vi "Mobility Calculator.vi"() -> ()   [LabVIEW 2011]
uses:
  <vilib>/picture/picture.llb/Draw True-Color Pixmap.vi
panel:
  in  "Blank Button":bool
  in  "Refresh Button":bool
  in  "tick mark length":i16=4
  in  "constant coordinate":i16=10
  out "picture":picture
  in  "scale definition":T1={"coordinate 1"=5, "value 1"=0.0, "coordinate 2"=50, "value 2"=10.0, "log"=FALSE, "fmt and prec"={"format"=enum."Decimal", "precision"=0}} {"value 2" format="%0.2f"; "value 1" format="%0.2f"}
  in  "scale attributes":T2={"horizontal"=FALSE, "left/top"=FALSE, "draw bar"=TRUE, "line color"=255, "text color"=0}
  out "2D Picture 2":picture
  out "Array 6":dbl[][](array[numeric])
  out "Cluster":T3
  out "Array 5":dbl[](array[numeric])
  out "Array 4":dbl[](array[numeric])
  out "Array 3":dbl[](array[numeric])
  out "Numeric 2":dbl
  out "Numeric":dbl
  out "2D Picture":picture
  in  "Path 3":path
  in  "Slide":dbl(slide) step=1.0 scale=-1.0..142.0 scale format="%#_1p"
  out "New Mobility":dbl
  out "Array 2":dbl[](array[numeric])
  out "Array":dbl[](array[numeric])
  in  "Width new":dbl
  in  "Length new":dbl
  in  "Dielectric (d) new":dbl
  in  "Save Changes?":bool
  out "Index":dbl
  out "String":string
  in  "Path 2":path
  in  "Down Button":bool
  in  "Up Button":bool
  in  "Previous Button":bool
  in  "Next Button":bool
  in  "Cancel Button":bool
  in  "NumPts":dbl=5.0
  out "XY Graph":cluster{dbl[], dbl[]}[](graph)
  out "Dielectric (d)":dbl
  out "Width":dbl
  out "Length":dbl
  out "Table Control 2":string[][](table)
  out "Table Control":string[][](table)
  in  "Row Start":dbl=20.0
  in  "Path":path
  out "Mobility":dbl
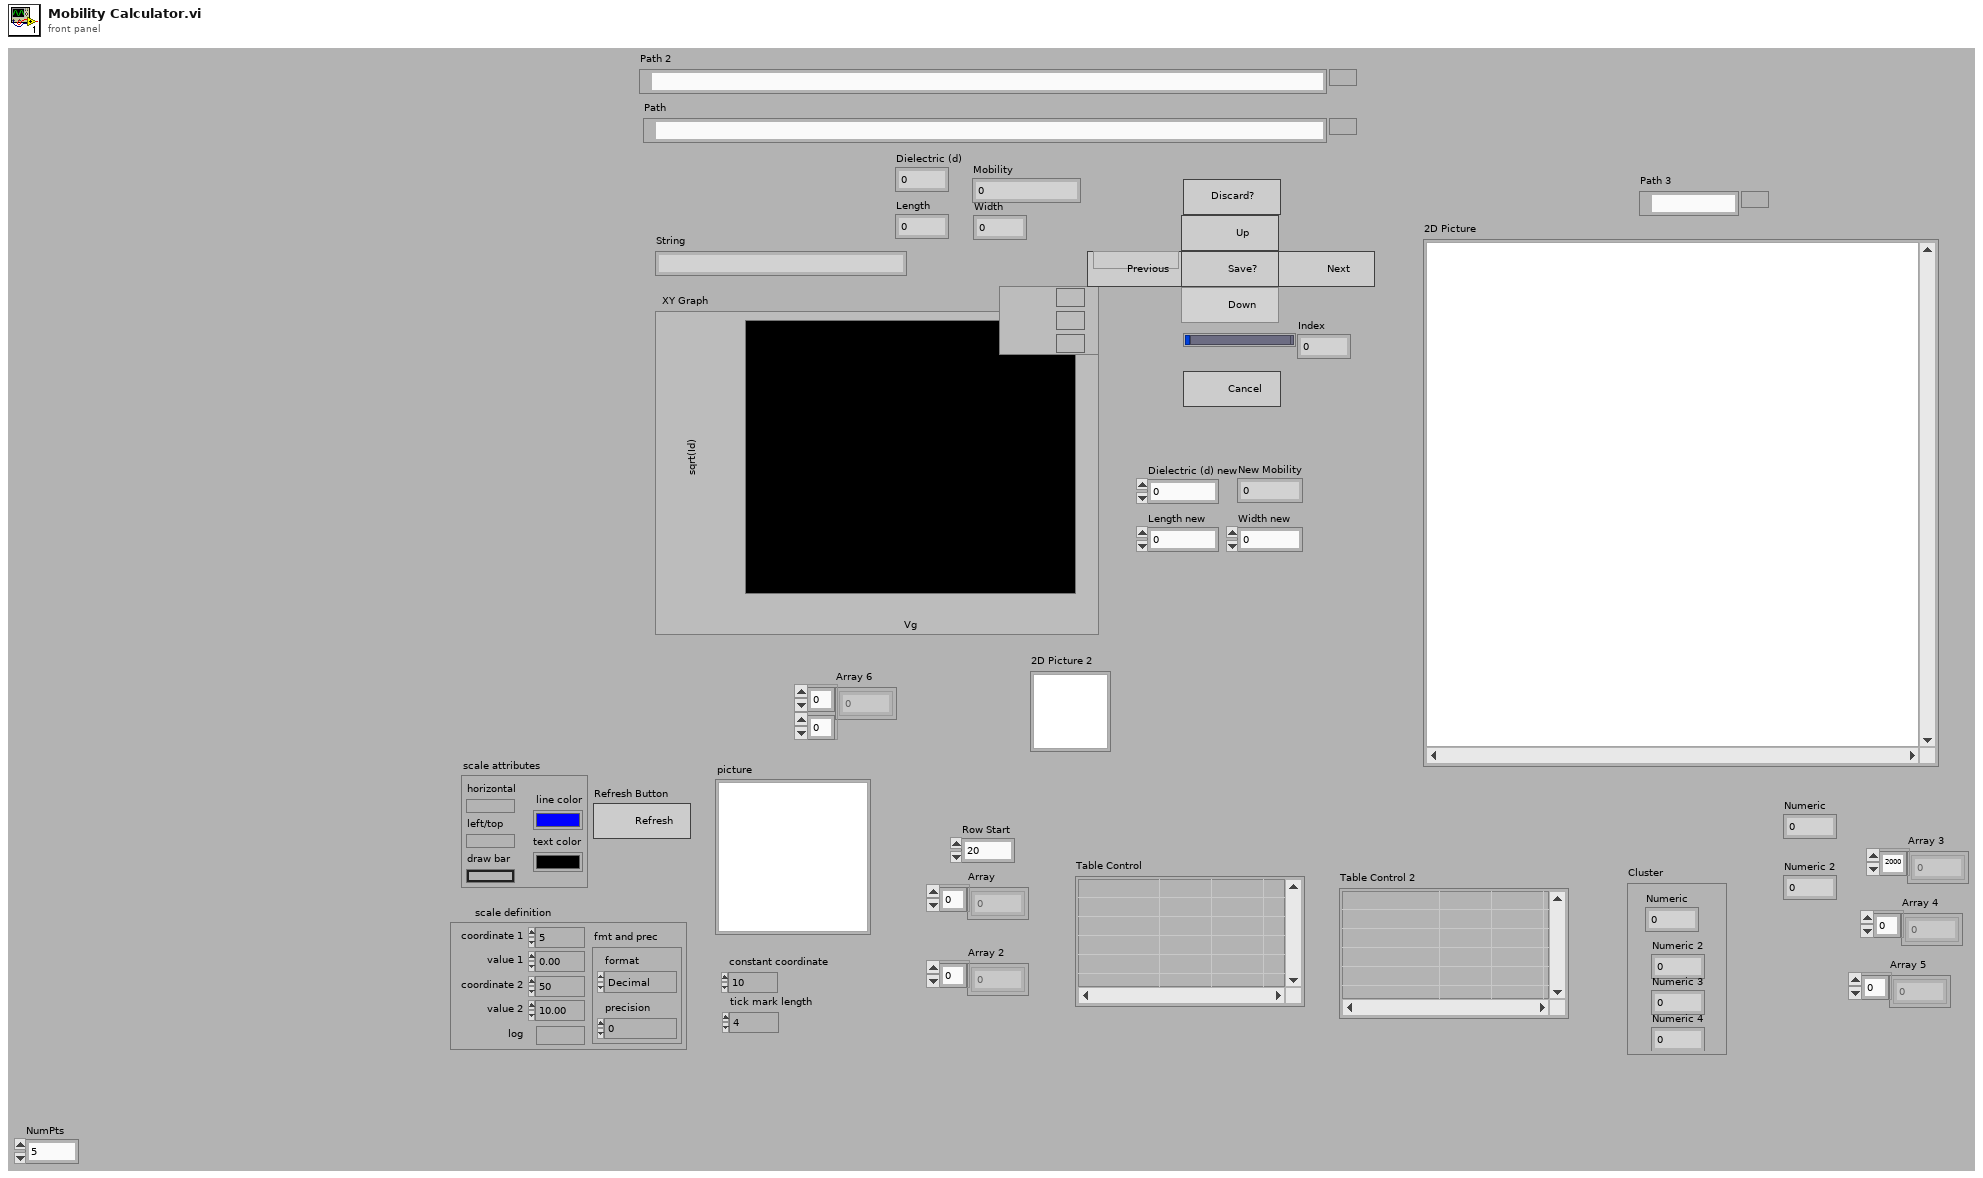
[diagram p1: front panel]
types:
  T1 = cluster{"coordinate 1":i16, "value 1":dbl, "coordinate 2":i16, "value 2":dbl, "log":bool, "fmt and prec":cluster{"format":enum8{"Decimal", "Scientific", "Engineering", "Binary", "Octal", "Hex"}, "precision":u8}}
  T2 = cluster{"horizontal":bool, "left/top":bool, "draw bar":bool, "line color":u32, "text color":u32}
  T3 = cluster{"Numeric":dbl, "Numeric 2":dbl, "Numeric 3":dbl, "Numeric 4":dbl}
  T4 = cluster{"[0]":cluster{dbl[], dbl[]}, "[1]":cluster{dbl[], dbl[]}, "[2]":cluster{dbl[], dbl[]}, "[3]":cluster{dbl[], dbl[]}, "[4]":cluster{dbl[], dbl[]}, "[5]":cluster{dbl[], dbl[]}, "[6]":cluster{dbl[], dbl[]}, "[7]":cluster{dbl[], dbl[]}, "[8]":cluster{dbl[], dbl[]}}
  T5 = typedef "imagedata.ctl" = cluster{"image type":i32, "image depth":i32, "image":u8[], "mask":u8[], "colors":u32[], "Rectangle":cluster{"left":i16, "top":i16, "right":i16, "bottom":i16}}
  T6 = cluster{"left":i16, "top":i16, "right":i16, "bottom":i16}
  T7 = cluster{"image type":i32, "image depth":i32, "image":u8[], "mask":u8[], "colors":u32[], cluster{dbl, dbl, dbl, dbl}}
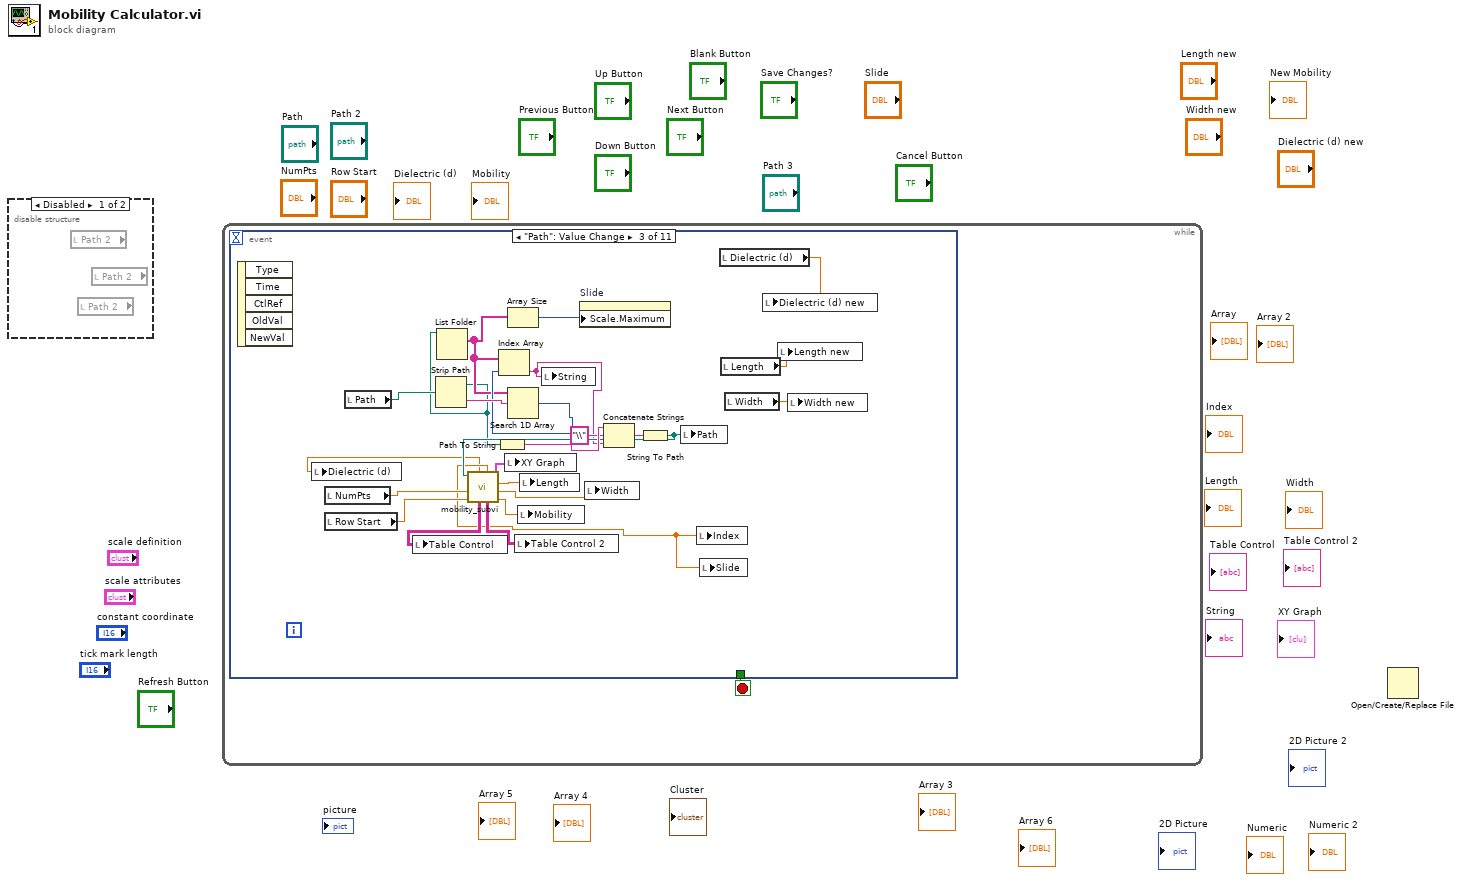
[diagram p0: block diagram]
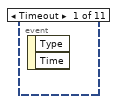
[diagram p3: hidden frame]
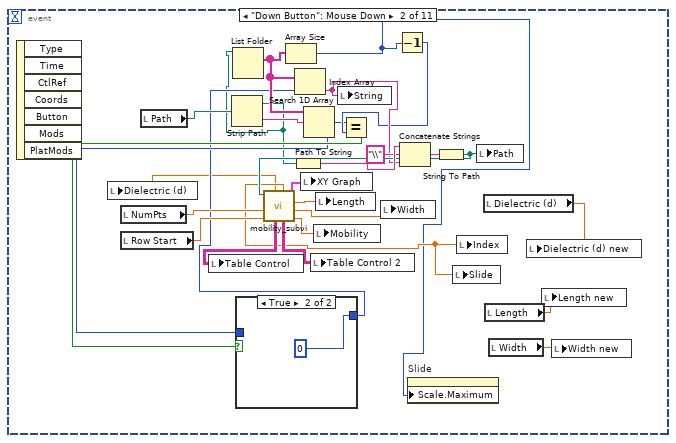
[diagram p4: hidden frame]
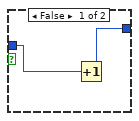
[diagram p5: hidden frame]
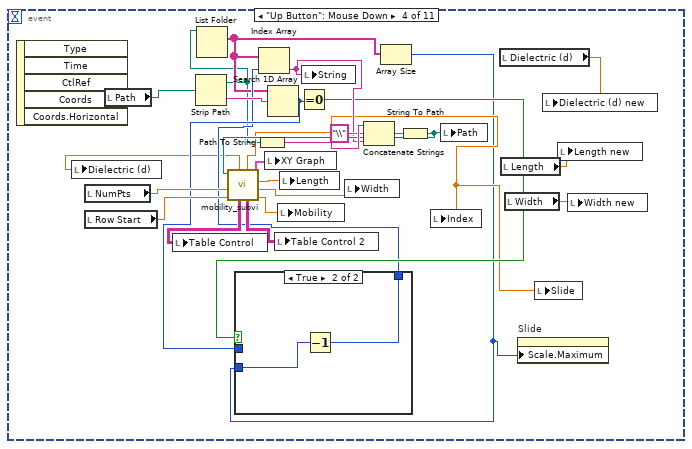
[diagram p6: hidden frame]
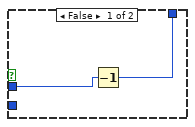
[diagram p7: hidden frame]
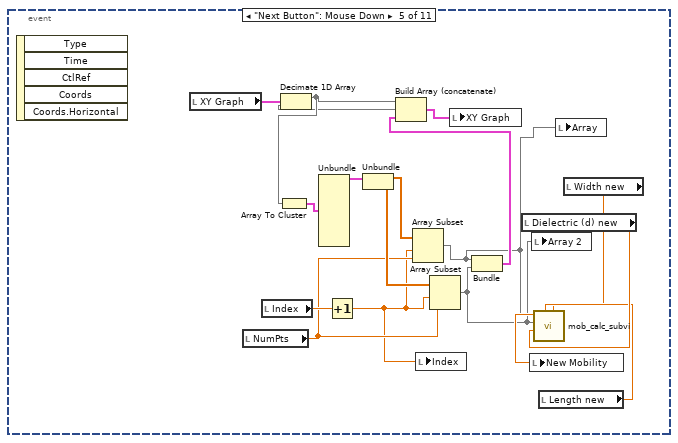
[diagram p8: hidden frame]
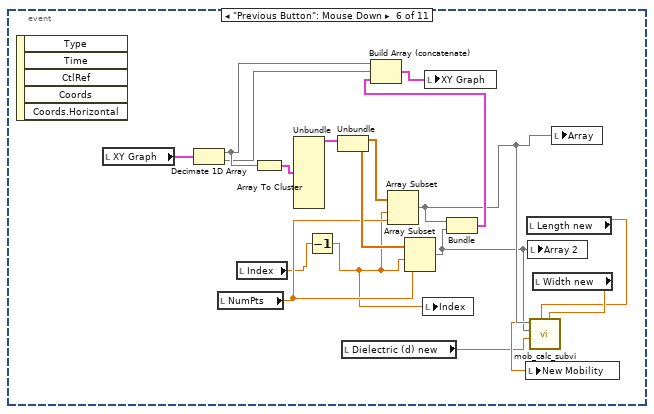
[diagram p9: hidden frame]
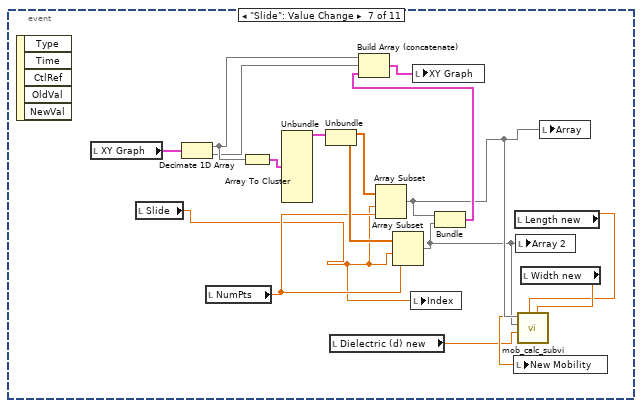
[diagram p10: hidden frame]
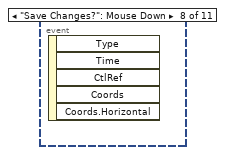
[diagram p11: hidden frame]
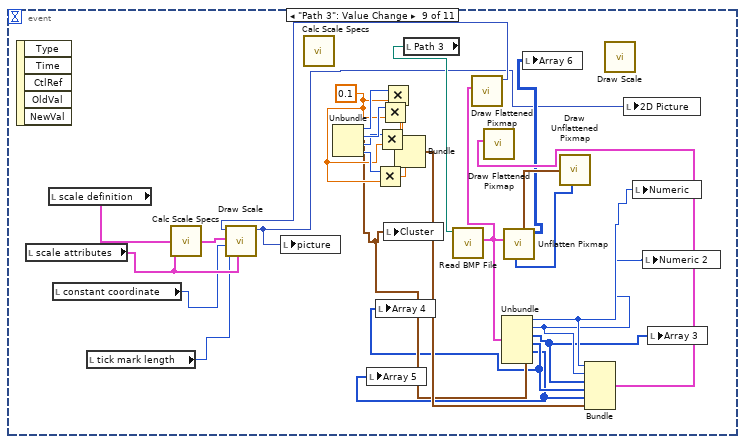
[diagram p12: hidden frame]
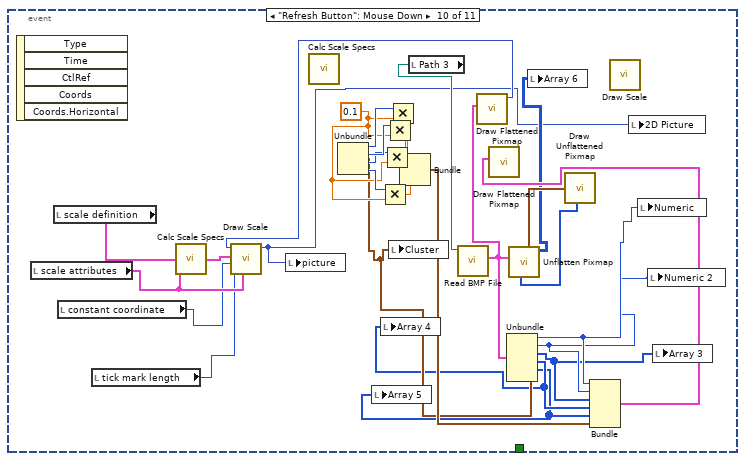
[diagram p13: hidden frame]
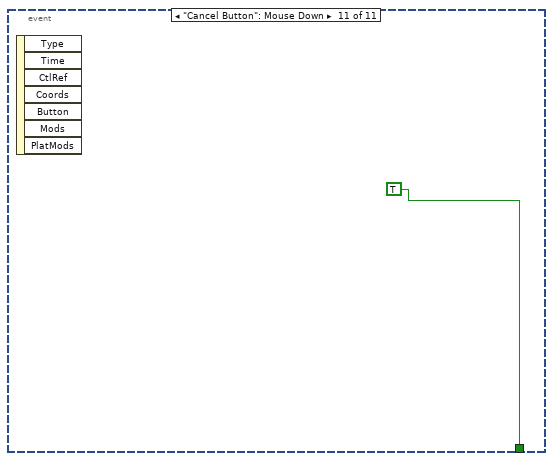
[diagram p14: hidden frame]
diagram:
  n1 = disable-structure shown="Disabled" {
    frame Disabled {
      n2 = local read "Path 2"() -> ()  [unwired: 1 out]
      n3 = local read "Path 2"() -> ()  [unwired: 1 out]
      n4 = local read "Path 2"() -> ()  [unwired: 1 out]
    }
    frame Enabled {
    }
  }
  n5 = while {
    stop <- w1 stop-if-true
    n6 = event shown="[2] \"Path\": Value Change" {
      selector: _ -> [_ _ _ _ _ _ _ _ _ _ _]
      dyn-events: _ -> [_ _ _ _ _ _ _ _ _ _ _]
      timeout: _ -> [_ _ _ _ _ _ _ _ _ _ _]
      tunnel: [_ _ _ _ _ _ _ _ _ _ TRUE] -> w1
      event Timeout {
        n7 = event-data() -> ()  [unwired: 1 in, 2 out]
      }
      event "Down Button": Mouse Down {
        n8 = event-data() -> ()  [unwired: 1 in, 7 out]
        n9 = local read "NumPts"() -> (w22:dbl)
        n10 = local read "Row Start"() -> (w21:dbl)
        n11 = local read "Path"() -> (w28:path)
        n12 = Strip Path(path=w28) -> (stripped path=w2:path, name=w26:string)
        n13 = List Folder(path=w2) -> (filenames=w13:string[])  [unwired: 3 in, 3 out]
        n14 = Array Size(array=w13) -> (size(s)=w4:i32)
        n15 = Path To String(path=w2) -> (string=w27:string)
        n16 = Search 1D Array(1D array=w13, element=w26) -> (index of element=w10:i32)  [unwired: 1 in]
        n17 = Decrement(x=w4) -> (x-1=w11:i32)
        n18 = Equal?(x=w10, y=w11) -> (x = y?=w12:bool)
        n19 = case shown="True" w12 {
          tunnel: w10 -> [w30 _]
          tunnel: [w29 0] -> w9
          frame False {
            n20 = Increment(x=w30) -> (x+1=w29:i32)
          }
          frame True {
          }
        }
        n21 = Index Array(array=w13, index=w9) -> (element=w14:string)
        n22 = local write "String"(w14) -> ()
        n23 = Concatenate Strings(w27, "\\", w14) -> (w25:string)
        n24 = property on="Slide" class="Slide (strict)"("Scale.Maximum"=w4) -> ()  [unwired: 2 in, 2 out]
        n25 = String To Path(string=w25) -> (path=w23:path)
        n26 = call "mobility_subvi.vi"("Row Start"=w21, "NumPts"=w22, "Path"=w23) -> ("Mobility"=w15:dbl, "Width"=w16:dbl, "Length"=w17:dbl, "XY Graph"=w18:cluster{dbl[], dbl[]}[], "Table Control 2"=w19:string[][], "Index"=w5:dbl, "Table Control"=w20:string[][], "Dielectric (d)"=w3:dbl)  [unwired: 1 in]
        n27 = local write "Dielectric (d)"(w3) -> ()
        n28 = local write "Table Control"(w20) -> ()
        n29 = local write "XY Graph"(w18) -> ()
        n30 = local write "Table Control 2"(w19) -> ()
        n31 = local write "Mobility"(w15) -> ()
        n32 = local write "Length"(w17) -> ()
        n33 = local write "Width"(w16) -> ()
        n34 = local write "Slide"(w5) -> ()
        n35 = local write "Index"(w5) -> ()
        n36 = local write "Path"(w23) -> ()
        n37 = local read "Dielectric (d)"() -> (w8:dbl)
        n38 = local read "Length"() -> (w7:dbl)
        n39 = local read "Width"() -> (w6:dbl)
        n40 = local write "Dielectric (d) new"(w8) -> ()
        n41 = local write "Length new"(w7) -> ()
        n42 = local write "Width new"(w6) -> ()
      }
      event "Path": Value Change {
        n43 = event-data() -> ()  [unwired: 1 in, 5 out]
        n44 = local read "NumPts"() -> (w49:dbl)
        n45 = local read "Row Start"() -> (w48:dbl)
        n46 = local read "Path"() -> (w55:path)
        n47 = Strip Path(path=w55) -> (stripped path=w32:path, name=w53:string)
        n48 = List Folder(path=w32) -> (filenames=w35:string[])  [unwired: 3 in, 3 out]
        n49 = Path To String(path=w32) -> (string=w54:string)
        n50 = Array Size(array=w35) -> (size(s)=w34:i32)
        n51 = Search 1D Array(1D array=w35, element=w53) -> (index of element=w40:i32)  [unwired: 1 in]
        n52 = Index Array(array=w35, index=w40) -> (element=w41:string)
        n53 = local write "String"(w41) -> ()
        n54 = property on="Slide" class="Slide (strict)"("Scale.Maximum"=w34) -> ()  [unwired: 2 in, 2 out]
        n55 = Concatenate Strings(w54, "\\", w41) -> (w52:string)
        n56 = String To Path(string=w52) -> (path=w50:path)
        n57 = call "mobility_subvi.vi"("Row Start"=w48, "NumPts"=w49, "Path"=w50) -> ("Mobility"=w42:dbl, "Width"=w43:dbl, "Length"=w44:dbl, "XY Graph"=w45:cluster{dbl[], dbl[]}[], "Table Control 2"=w46:string[][], "Index"=w36:dbl, "Table Control"=w47:string[][], "Dielectric (d)"=w33:dbl)  [unwired: 1 in]
        n58 = local write "Dielectric (d)"(w33) -> ()
        n59 = local write "Table Control"(w47) -> ()
        n60 = local write "XY Graph"(w45) -> ()
        n61 = local write "Table Control 2"(w46) -> ()
        n62 = local write "Mobility"(w42) -> ()
        n63 = local write "Length"(w44) -> ()
        n64 = local write "Width"(w43) -> ()
        n65 = local write "Path"(w50) -> ()
        n66 = local write "Index"(w36) -> ()
        n67 = local write "Slide"(w36) -> ()
        n68 = local read "Dielectric (d)"() -> (w39:dbl)
        n69 = local read "Length"() -> (w38:dbl)
        n70 = local read "Width"() -> (w37:dbl)
        n71 = local write "Dielectric (d) new"(w39) -> ()
        n72 = local write "Length new"(w38) -> ()
        n73 = local write "Width new"(w37) -> ()
      }
      event "Up Button": Mouse Down {
        n74 = event-data() -> ()  [unwired: 1 in, 5 out]
        n75 = local read "NumPts"() -> (w75:dbl)
        n76 = local read "Row Start"() -> (w74:dbl)
        n77 = local read "Path"() -> (w81:path)
        n78 = Strip Path(path=w81) -> (stripped path=w56:path, name=w79:string)
        n79 = List Folder(path=w56) -> (filenames=w63:string[])  [unwired: 3 in, 3 out]
        n80 = Path To String(path=w56) -> (string=w80:string)
        n81 = Search 1D Array(1D array=w63, element=w79) -> (index of element=w65:i32)  [unwired: 1 in]
        n82 = Equal To 0?(x=w65) -> (x = 0?=w66:bool)
        n83 = Array Size(array=w63) -> (size(s)=w58:i32)
        n84 = case shown="True" w66 {
          tunnel: w65 -> [w83 _]
          tunnel: [w82 w84] -> w64
          tunnel: w58 -> [_ w85]
          frame False {
            n85 = Decrement(x=w83) -> (x-1=w82:i32)
          }
          frame True {
            n86 = Decrement(x=w85) -> (x-1=w84:i32)
          }
        }
        n87 = Index Array(array=w63, index=w64) -> (element=w67:string)
        n88 = local write "String"(w67) -> ()
        n89 = Concatenate Strings(w80, "\\", w67) -> (w78:string)
        n90 = String To Path(string=w78) -> (path=w76:path)
        n91 = call "mobility_subvi.vi"("Row Start"=w74, "NumPts"=w75, "Path"=w76) -> ("Mobility"=w68:dbl, "Width"=w69:dbl, "Length"=w70:dbl, "XY Graph"=w71:cluster{dbl[], dbl[]}[], "Table Control 2"=w72:string[][], "Index"=w59:dbl, "Table Control"=w73:string[][], "Dielectric (d)"=w57:dbl)  [unwired: 1 in]
        n92 = local write "Dielectric (d)"(w57) -> ()
        n93 = local write "Table Control"(w73) -> ()
        n94 = local write "XY Graph"(w71) -> ()
        n95 = local write "Table Control 2"(w72) -> ()
        n96 = local write "Mobility"(w68) -> ()
        n97 = local write "Length"(w70) -> ()
        n98 = local write "Width"(w69) -> ()
        n99 = local write "Index"(w59) -> ()
        n100 = local write "Path"(w76) -> ()
        n101 = local read "Dielectric (d)"() -> (w62:dbl)
        n102 = local read "Length"() -> (w61:dbl)
        n103 = local read "Width"() -> (w60:dbl)
        n104 = property on="Slide" class="Slide (strict)"("Scale.Maximum"=w58) -> ()  [unwired: 2 in, 2 out]
        n105 = local write "Slide"(w59) -> ()
        n106 = local write "Dielectric (d) new"(w62) -> ()
        n107 = local write "Length new"(w61) -> ()
        n108 = local write "Width new"(w60) -> ()
      }
      event "Next Button": Mouse Down {
        n109 = event-data() -> ()  [unwired: 1 in, 5 out]
        n110 = local read "XY Graph"() -> (w97:cluster{dbl[], dbl[]}[])
        n111 = local read "NumPts"() -> (w98:dbl)
        n112 = local read "Index"() -> (w99:dbl)
        n113 = Decimate 1D Array(w97) -> (w93:cluster{dbl[], dbl[]}[], w92:cluster{dbl[], dbl[]}[])
        n114 = Array To Cluster(array=w93) -> (cluster=w103:T4)
        n115 = Unbundle(w103) -> ("[0]"=w102:cluster{dbl[], dbl[]})  [unwired: 8 out]
        n116 = Increment(x=w99) -> (x+1=w94:dbl)
        n117 = Unbundle(w102) -> (w101:dbl[], w100:dbl[])
        n118 = Array Subset(array=w101, index=w94, length=w98) -> (w90:dbl[])
        n119 = local write "Index"(w94) -> ()
        n120 = Array Subset(array=w100, index=w94, length=w98) -> (w89:dbl[])
        n121 = Bundle(w90, w89) -> (w96:cluster{dbl[], dbl[]})  [unwired: 1 in]
        n122 = Build Array (concatenate)(w93, w92, w96) -> (w95:cluster{dbl[], dbl[]}[])
        n123 = local write "XY Graph"(w95) -> ()
        n124 = local read "Dielectric (d) new"() -> (w88:dbl)
        n125 = local write "Array 2"(w89) -> ()
        n126 = local read "Length new"() -> (w87:dbl)
        n127 = local write "Array"(w90) -> ()
        n128 = local read "Width new"() -> (w86:dbl)
        n129 = call "mob_calc_subvi.vi"("Width"=w86, "Length"=w87, "Dielectric (d)"=w88, "Array 2"=w89, "Array"=w90) -> ("Mobility"=w91:dbl)  [unwired: 5 in, 1 out]
        n130 = local write "New Mobility"(w91) -> ()
      }
      event "Previous Button": Mouse Down {
        n131 = event-data() -> ()  [unwired: 1 in, 5 out]
        n132 = local read "XY Graph"() -> (w116:cluster{dbl[], dbl[]}[])
        n133 = Decimate 1D Array(w116) -> (w113:cluster{dbl[], dbl[]}[], w112:cluster{dbl[], dbl[]}[])
        n134 = local read "NumPts"() -> (w117:dbl)
        n135 = local read "Index"() -> (w111:dbl)
        n136 = Array To Cluster(array=w113) -> (cluster=w121:T4)
        n137 = Unbundle(w121) -> ("[0]"=w120:cluster{dbl[], dbl[]})  [unwired: 8 out]
        n138 = Decrement(x=w111) -> (x-1=w110:dbl)
        n139 = Unbundle(w120) -> (w119:dbl[], w118:dbl[])
        n140 = local read "Dielectric (d) new"() -> (w104:dbl)
        n141 = Array Subset(array=w119, index=w110, length=w117) -> (w109:dbl[])
        n142 = Array Subset(array=w118, index=w110, length=w117) -> (w108:dbl[])
        n143 = local write "Index"(w110) -> ()
        n144 = Bundle(w109, w108) -> (w115:cluster{dbl[], dbl[]})  [unwired: 1 in]
        n145 = Build Array (concatenate)(w113, w112, w115) -> (w114:cluster{dbl[], dbl[]}[])
        n146 = local write "XY Graph"(w114) -> ()
        n147 = local read "Length new"() -> (w105:dbl)
        n148 = local write "Array 2"(w108) -> ()
        n149 = local read "Width new"() -> (w106:dbl)
        n150 = call "mob_calc_subvi.vi"("Width"=w106, "Length"=w105, "Dielectric (d)"=w104, "Array 2"=w108, "Array"=w109) -> ("Mobility"=w107:dbl)  [unwired: 5 in, 1 out]
        n151 = local write "New Mobility"(w107) -> ()
        n152 = local write "Array"(w109) -> ()
      }
      event "Slide": Value Change {
        n153 = event-data() -> ()  [unwired: 1 in, 5 out]
        n154 = local read "XY Graph"() -> (w133:cluster{dbl[], dbl[]}[])
        n155 = local read "Slide"() -> (w122:dbl)
        n156 = Decimate 1D Array(w133) -> (w130:cluster{dbl[], dbl[]}[], w129:cluster{dbl[], dbl[]}[])
        n157 = local read "NumPts"() -> (w134:dbl)
        n158 = Array To Cluster(array=w130) -> (cluster=w138:T4)
        n159 = Unbundle(w138) -> ("[0]"=w137:cluster{dbl[], dbl[]})  [unwired: 8 out]
        n160 = Unbundle(w137) -> (w136:dbl[], w135:dbl[])
        n161 = local read "Dielectric (d) new"() -> (w123:dbl)
        n162 = Array Subset(array=w136, index=w122, length=w134) -> (w128:dbl[])
        n163 = Array Subset(array=w135, index=w122, length=w134) -> (w127:dbl[])
        n164 = local write "Index"(w122) -> ()
        n165 = Bundle(w128, w127) -> (w132:cluster{dbl[], dbl[]})  [unwired: 1 in]
        n166 = Build Array (concatenate)(w130, w129, w132) -> (w131:cluster{dbl[], dbl[]}[])
        n167 = local write "XY Graph"(w131) -> ()
        n168 = local read "Length new"() -> (w124:dbl)
        n169 = local write "Array 2"(w127) -> ()
        n170 = local read "Width new"() -> (w125:dbl)
        n171 = call "mob_calc_subvi.vi"("Width"=w125, "Length"=w124, "Dielectric (d)"=w123, "Array 2"=w127, "Array"=w128) -> ("Mobility"=w126:dbl)  [unwired: 5 in, 1 out]
        n172 = local write "New Mobility"(w126) -> ()
        n173 = local write "Array"(w128) -> ()
      }
      event "Save Changes?": Mouse Down {
        n174 = event-data() -> ()  [unwired: 1 in, 5 out]
      }
      event "Path 3": Value Change {
        w161 = 0.1
        n175 = event-data() -> ()  [unwired: 1 in, 5 out]
        n176 = local read "scale attributes"() -> (w141:T2)
        n177 = local read "scale definition"() -> (w142:T1)
        n178 = local read "constant coordinate"() -> (w140:i16)
        n179 = local read "tick mark length"() -> (w139:i16)
        n180 = call <vilib>:"Calc Scale Specs.vi"("scale definition"=w142, "scale attributes"=w141) -> ("scale specs"=w153:cluster{"coordinate":i16, "label":string}[])  [unwired: 7 in]
        n181 = call <vilib>:"Calc Scale Specs.vi"() -> ()  [unwired: 9 in, 1 out]
        n182 = local read "Path 3"() -> (w144:path)
        n183 = call <vilib>:"Read BMP File.vi"("path to BMP file"=w144) -> ("image data"=w154:T5)  [unwired: 8 in, 2 out]
        n184 = call <vilib>:"Draw Flattened Pixmap.vi"("image data"=w154) -> ("new picture"=w148:picture)  [unwired: 8 in]
        n185 = call <vilib>:"Draw Scale.vi"("scale attributes"=w141, "tick length(3)"=w139, "constant coordinate"=w140, "scale specs"=w153, "picture"=w148) -> ("new picture"=w143:picture)  [unwired: 6 in]
        n186 = local write "picture"(w143) -> ()
        n187 = Unbundle(w154) -> ("image type"=w151:i32, "image depth"=w150:i32, "image"=w149:u8[], "mask"=w146:u8[], "colors"=w145:u32[], "Rectangle"=w147:T6)
        n188 = Unbundle(w147) -> ("left"=w165:i16, "top"=w164:i16, "right"=w163:i16, "bottom"=w162:i16)
        n189 = local write "Array 5"(w145) -> ()
        n190 = Multiply(x=w162, y=w161) -> (x*y=w157:dbl)
        n191 = local write "Array 4"(w146) -> ()
        n192 = Multiply(x=w163, y=w161) -> (x*y=w158:dbl)
        n193 = Multiply(x=w164, y=w161) -> (x*y=w159:dbl)
        n194 = Multiply(x=w165, y=w161) -> (x*y=w160:dbl)
        n195 = local write "Cluster"(w147) -> ()
        n196 = Bundle(w160, w159, w158, w157) -> (w156:cluster{dbl, dbl, dbl, dbl})  [unwired: 1 in]
        n197 = call <vilib>:"Unflatten Pixmap.vi"("image data"=w154) -> ("24-bit pixmap"=w152:u32[][], "top left"=w166:cluster{"x":i16, "y":i16}, "mask"=w167:u8[])  [unwired: 4 in, 4 out]
        n198 = local write "Array 6"(w152) -> ()
        n199 = call-poly <vilib>:"Draw Unflattened Pixmap.vi"("top left point(0, 0)"=w166, "mask"=w167) -> ()  [unwired: 7 in, 1 out]
        n200 = Bundle("image type"=w151, "image depth"=w150, "image"=w149, "mask"=w146, "colors"=w145, w156) -> (w155:T7)  [unwired: 1 in]
        n201 = call <vilib>:"Draw Flattened Pixmap.vi"("image data"=w155) -> ()  [unwired: 8 in, 1 out]
        n202 = call <vilib>:"Draw Scale.vi"() -> ()  [unwired: 11 in, 1 out]
        n203 = local write "2D Picture"(w143) -> ()
        n204 = local write "Numeric"(w151) -> ()
        n205 = local write "Numeric 2"(w150) -> ()
        n206 = local write "Array 3"(w149) -> ()
      }
      event "Refresh Button": Mouse Down {
        w190 = 0.1
        n207 = event-data() -> ()  [unwired: 1 in, 5 out]
        n208 = local read "scale attributes"() -> (w170:T2)
        n209 = local read "scale definition"() -> (w171:T1)
        n210 = local read "constant coordinate"() -> (w169:i16)
        n211 = local read "tick mark length"() -> (w168:i16)
        n212 = call <vilib>:"Calc Scale Specs.vi"("scale definition"=w171, "scale attributes"=w170) -> ("scale specs"=w182:cluster{"coordinate":i16, "label":string}[])  [unwired: 7 in]
        n213 = call <vilib>:"Calc Scale Specs.vi"() -> ()  [unwired: 9 in, 1 out]
        n214 = local read "Path 3"() -> (w173:path)
        n215 = call <vilib>:"Read BMP File.vi"("path to BMP file"=w173) -> ("image data"=w183:T5)  [unwired: 8 in, 2 out]
        n216 = call <vilib>:"Draw Flattened Pixmap.vi"("image data"=w183) -> ("new picture"=w177:picture)  [unwired: 8 in]
        n217 = call <vilib>:"Draw Scale.vi"("scale attributes"=w170, "tick length(3)"=w168, "constant coordinate"=w169, "scale specs"=w182, "picture"=w177) -> ("new picture"=w172:picture)  [unwired: 6 in]
        n218 = local write "picture"(w172) -> ()
        n219 = Unbundle(w183) -> ("image type"=w180:i32, "image depth"=w179:i32, "image"=w178:u8[], "mask"=w175:u8[], "colors"=w174:u32[], "Rectangle"=w176:T6)
        n220 = Unbundle(w176) -> ("left"=w194:i16, "top"=w193:i16, "right"=w192:i16, "bottom"=w191:i16)
        n221 = local write "Array 5"(w174) -> ()
        n222 = Multiply(x=w191, y=w190) -> (x*y=w186:dbl)
        n223 = local write "Array 4"(w175) -> ()
        n224 = Multiply(x=w192, y=w190) -> (x*y=w187:dbl)
        n225 = Multiply(x=w193, y=w190) -> (x*y=w188:dbl)
        n226 = Multiply(x=w194, y=w190) -> (x*y=w189:dbl)
        n227 = local write "Cluster"(w176) -> ()
        n228 = Bundle(w189, w188, w187, w186) -> (w185:cluster{dbl, dbl, dbl, dbl})  [unwired: 1 in]
        n229 = call <vilib>:"Unflatten Pixmap.vi"("image data"=w183) -> ("24-bit pixmap"=w181:u32[][], "top left"=w195:cluster{"x":i16, "y":i16}, "mask"=w196:u8[])  [unwired: 4 in, 4 out]
        n230 = local write "Array 6"(w181) -> ()
        n231 = call-poly <vilib>:"Draw Unflattened Pixmap.vi"("top left point(0, 0)"=w195, "mask"=w196) -> ()  [unwired: 7 in, 1 out]
        n232 = Bundle("image type"=w180, "image depth"=w179, "image"=w178, "mask"=w175, "colors"=w174, w185) -> (w184:T7)  [unwired: 1 in]
        n233 = call <vilib>:"Draw Flattened Pixmap.vi"("image data"=w184) -> ()  [unwired: 8 in, 1 out]
        n234 = call <vilib>:"Draw Scale.vi"() -> ()  [unwired: 11 in, 1 out]
        n235 = local write "2D Picture"(w172) -> ()
        n236 = local write "Numeric"(w180) -> ()
        n237 = local write "Numeric 2"(w179) -> ()
        n238 = local write "Array 3"(w178) -> ()
      }
      event "Cancel Button": Mouse Down {
        n239 = event-data() -> ()  [unwired: 1 in, 7 out]
      }
    }
  }
  n240 = Open/Create/Replace File() -> ()  [unwired: 6 in, 3 out]
